vi "menu-Config menu items.vi"() -> (2 "item tags":string[](array[string]), 3 "item names":string[](array[string]))   [LabVIEW 2017]
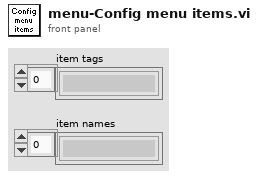
[diagram p1: front panel]
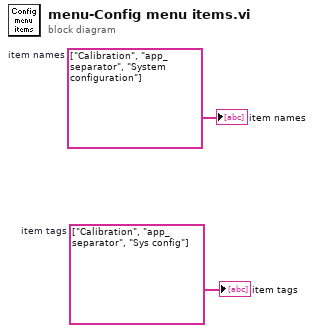
[diagram p0: block diagram]
diagram:
  w2 = string[] ["Calibration", "app_separator", "System configuration"]  # item names
  w1 = string[] ["Calibration", "app_separator", "Sys config"]  # item tags
  "item names" <- w2
  "item tags" <- w1
